vi "Update UI.vi"(8 "error in (no error)":errorcluster, 10 "DataExchange":T1, 11 "Controller Template in":refnum<class "FlatFieldUI.lvclass">) -> (0 "error out":errorcluster, 3 "Controller Template out":refnum<class "FlatFieldUI.lvclass">)   [LabVIEW 2020, in "FlatField.lvlib" / "FlatFieldUI.lvlib" / "FlatFieldUI.lvclass"]
uses:
  FlatFieldUI.lvclass
  Hardware Abstraction Layer/Component/Device/Device/DataExchange.ctl
  FlatFieldUI.lvclass/FlatFieldUI.ctl
  <vilib>/vision/Image Controls.llb/IMAQ Image.ctl
  Interface/DataListener/DataListener.lvclass
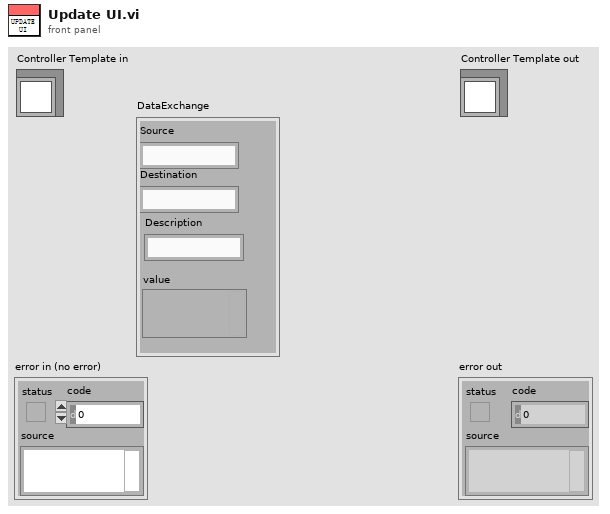
[diagram p1: front panel]
types:
  T1 = typedef "DataListener.lvclass/DataExchange.ctl" = cluster{"Source":string, "Destination":string, "Description":string, "value":variant}
  T2 = typedef "IMAQ Image.ctl" = refnum<image>
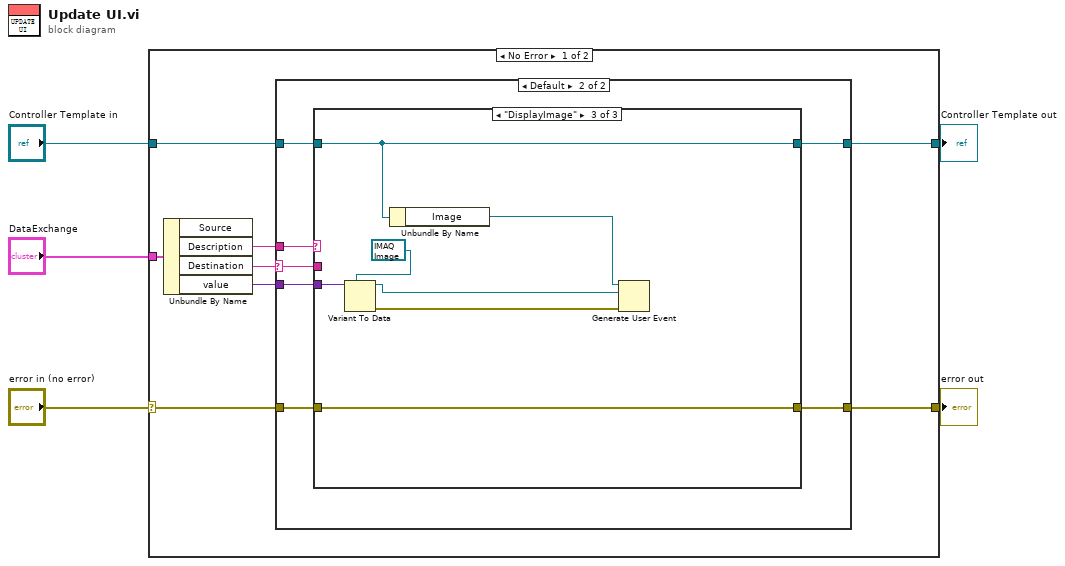
[diagram p0: block diagram]
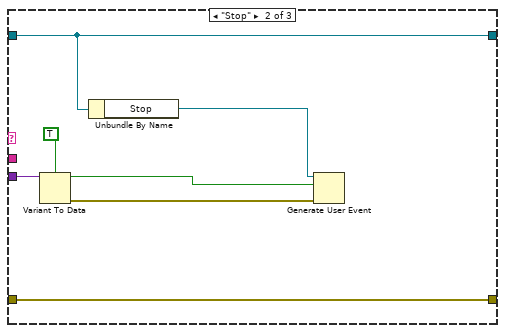
[diagram p4: hidden frame]
diagram:
  n1 = case shown="No Error" "error in (no error)" {
    selector: "error in (no error)" -> [w8 w40]
    tunnel: [w7 w40] -> w4
    tunnel: [w9 w39] -> w2
    tunnel: "Controller Template in" -> [w10 w39]
    tunnel: "DataExchange" -> [w13 _]
    frame No Error {
      n2 = Unbundle By Name(w13) -> ("Description"=w11:string, "Destination"=w6:string, "value"=w12:variant)  [unwired: 1 out]
      n3 = case shown="Default" w6 {
        selector: w6 -> [_ w16]
        tunnel: w12 -> [_ w22]
        tunnel: w11 -> [_ w21]
        tunnel: w10 -> [w15 w20]
        tunnel: [w15 w19] -> w9
        tunnel: w8 -> [w14 w18]
        tunnel: [w14 w17] -> w7
        frame "duplicate this case" {
        }
        frame Default {
          n4 = case shown="\"DisplayImage\"" w21 {
            tunnel: w22 -> [_ w31 w38]
            tunnel: [w24 w26 w35] -> w19
            tunnel: w20 -> [w24 w26 w35]
            tunnel: [w23 w25 w34] -> w17
            tunnel: w18 -> [w23 w25 w34]
            tunnel: w16 -> [_ _ _]
            frame Default {
            }
            frame "Stop" {
              n5 = Variant To Data(type=TRUE, Variant=w31) -> (data=w29:bool, error out=w27:errorcluster)  [unwired: 1 in]
              n6 = Unbundle By Name(w26) -> ("Stop"=w30:refnum<user-event>)
              n7 = Generate User Event(user event=w30, event data cluster=w29, error in=w27) -> ()  [unwired: 1 in, 2 out]
            }
            frame "DisplayImage" {
              n8 = Variant To Data(type=T2 refnum ("event data"), Variant=w38) -> (data=w32:T2, error out=w36:errorcluster)  [unwired: 1 in]
              n9 = Unbundle By Name(w35) -> ("Image"=w37:refnum<user-event>)
              n10 = Generate User Event(user event=w37, event data cluster=w32, error in=w36) -> ()  [unwired: 1 in, 2 out]
            }
          }
        }
      }
    }
    frame Error {
    }
  }
  "error out" <- w4
  "Controller Template out" <- w2
